vi "CF_TC_to_DSC.vi"(8 "error in (no error)":errorcluster, 9 "calibration string":string, 10 "description string":string, 11 "dbl":dbl[](array[numeric])) -> (0 "error out":errorcluster)   [LabVIEW 2013]
panel:
  in  "calibration string var":refnum<k21>="ni.var.psp://housesoftheholy/Leiden CF900/CF_TC_calibration"
  in  "description string var":refnum<k21>="ni.var.psp://housesoftheholy/Leiden CF900/CF_TC_description"
  in  "dbl var":refnum<k21>[](array[refnum])=["ni.var.psp://housesoftheholy/Leiden CF900/Leiden CF TC/CF TC R0", "ni.var.psp://housesoftheholy/Leiden CF900/Leiden CF TC/CF TC R1", "ni.var.psp://housesoftheholy/Leiden CF900/Leiden CF TC/CF TC R2", "ni.var.psp://housesoftheholy/Leiden CF900/Leiden CF TC/CF TC R3", "ni.var.psp://housesoftheholy/Leiden CF900/Leiden CF TC/CF TC R4", "ni.var.psp://housesoftheholy/Leiden CF900/Leiden CF TC/CF TC R5", "ni.var.psp://housesoftheholy/Leiden CF900/Leiden CF TC/CF TC R6", "ni.var.psp://housesoftheholy/Leiden CF900/Leiden CF TC/CF TC R7", "ni.var.psp://housesoftheholy/Leiden CF900/Leiden CF TC/CF TC T0", "ni.var.psp://housesoftheholy/Leiden CF900/Leiden CF TC/CF TC T1", "ni.var.psp://housesoftheholy/Leiden CF900/Leiden CF TC/CF TC T2", "ni.var.psp://housesoftheholy/Leiden CF900/Leiden CF TC/CF TC T3", "ni.var.psp://housesoftheholy/Leiden CF900/Leiden CF TC/CF TC T4", "ni.var.psp://housesoftheholy/Leiden CF900/Leiden CF TC/CF TC T5", "ni.var.psp://housesoftheholy/Leiden CF900/Leiden CF TC/CF TC T6", "ni.var.psp://housesoftheholy/Leiden CF900/Leiden CF TC/CF TC T7", "ni.var.psp://housesoftheholy/Leiden CF900/Leiden CF TC/CF TC I0", "ni.var.psp://housesoftheholy/Leiden CF900/Leiden CF TC/CF TC I1", "ni.var.psp://housesoftheholy/Leiden CF900/Leiden CF TC/CF TC I2", "ni.var.psp://housesoftheholy/Leiden CF900/Leiden CF TC/CF TC I3"]
  # "CF TC to DSC"
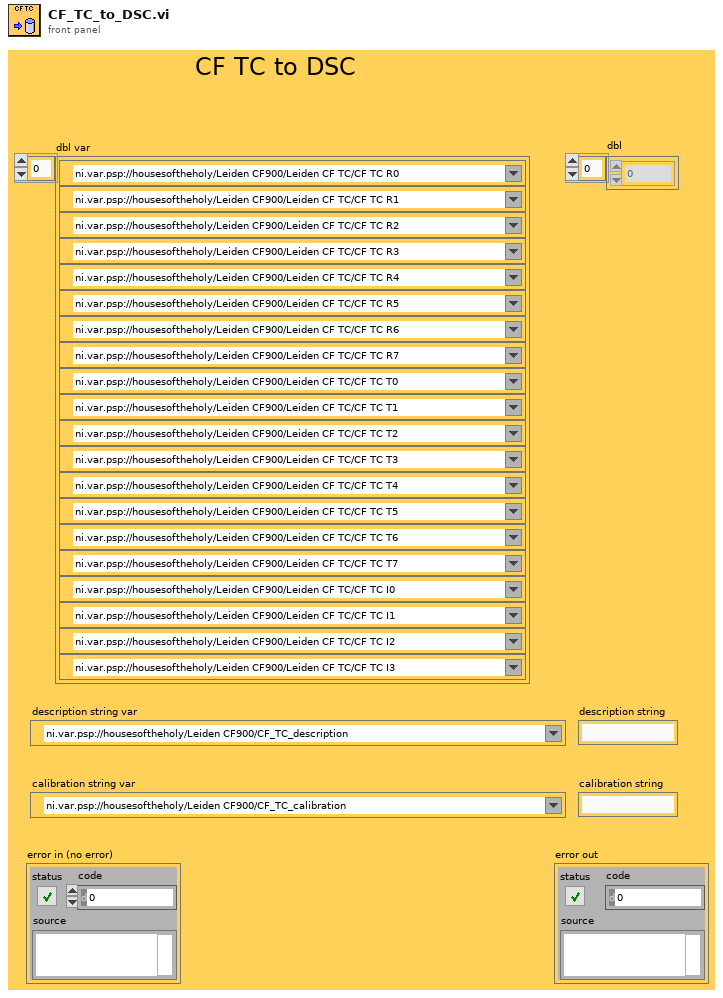
[diagram p1: front panel]
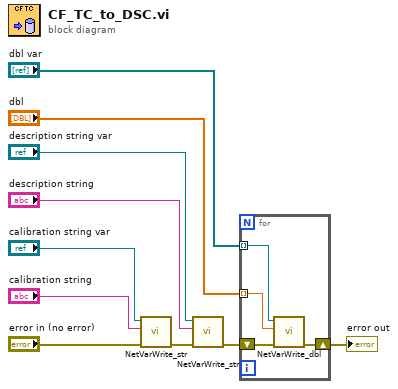
[diagram p0: block diagram]
diagram:
  n1 = call "NetVarWrite_str.vi"("error in (no error)"="error in (no error)", "String"="calibration string", "Refnum in"="calibration string var") -> ("error out"=w5:errorcluster)  [unwired: 8 in]
  n2 = call "NetVarWrite_str.vi"("error in (no error)"=w5, "String"="description string", "Refnum in"="description string var") -> ("error out"=w3:errorcluster)  [unwired: 8 in]
  n3 = for {
    tunnel: "dbl var" -> [w14] mode=indexing
    tunnel: "dbl" -> [w13] mode=indexing
    shift-right: [w11] -> w10
    shift-left: w3 -> [w12]
    n4 = call "NetVarWrite_dbl.vi"("error in (no error)"=w12, "Numeric"=w13, "Refnum in"=w14) -> ("error out"=w11:errorcluster)  [unwired: 8 in]
  }
  "error out" <- w10
